vi "setGPIOLineModeToInput.vi"(8 "error in (no error)":errorcluster, 10 "GPIO line":string, 11 "IMAQdx Session in":T1) -> (0 "error out":errorcluster, 3 "IMAQdx Session out":T1)   [LabVIEW 2017]
doc: "Set specified GPIO line on USB3 video camera as an input to use for triggering"
uses:
  <vilib>/userdefined/High Color/IMAQdx.ctl
  <resource>/objmgr/imaqdx.rc
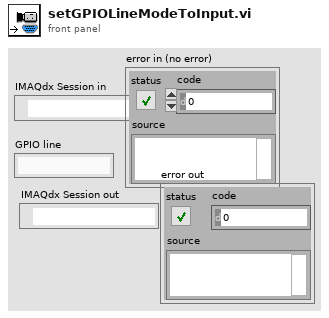
[diagram p1: front panel]
types:
  T1 = typedef "IMAQdx.ctl" = refnum<k21>
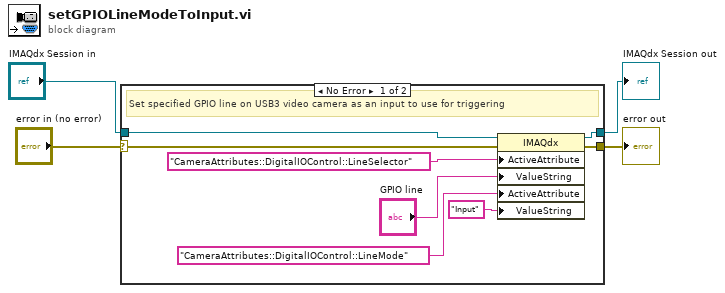
[diagram p0: block diagram]
diagram:
  n1 = case shown="No Error" "error in (no error)" {
    selector: "error in (no error)" -> [w7 w14]
    tunnel: [w8 w14] -> w4
    tunnel: "IMAQdx Session in" -> [w6 w13]
    tunnel: [w5 w13] -> w1
    frame No Error {
      # "Set specified GPIO line on USB3 video camera as an input to use for triggering"
      n2 = property class="IMAQdx"(reference=w6, error in=w7, "ActiveAttribute"="CameraAttributes::DigitalIOControl::LineSelector", "ValueString"="GPIO line", "ActiveAttribute"="CameraAttributes::DigitalIOControl::LineMode", "ValueString"="Input") -> (reference out=w5:T1, error out=w8:errorcluster)
    }
    frame Error {
    }
  }
  "error out" <- w4
  "IMAQdx Session out" <- w1
